vi "Send Message.vi"(7 "Data DVR":refnum<data-value>, 8 "Error In":errorcluster, 11 "Notify Only in":refnum<class "Notify Only.lvclass">) -> (0 "Error Out":errorcluster, 3 "Notify Only out":refnum<class "Notify Only.lvclass">)   [LabVIEW 2023, in "Notify Only.lvclass"]
uses:
  Notify Only.lvclass
  Data/Data.lvclass
  Controls/User Event Operations.ctl
  Notify Only.lvclass/Notify Only.ctl
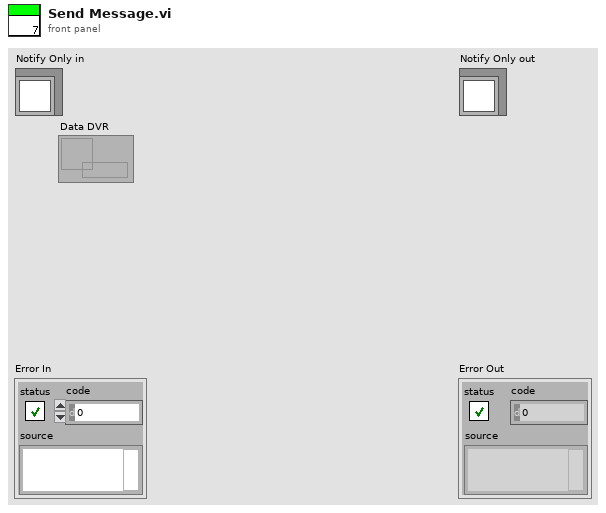
[diagram p1: front panel]
types:
  T1 = typedef "User Event Operations.ctl" = enum16{"Obtain", "Generate", "Destroy"}
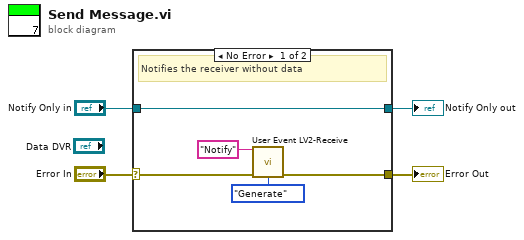
[diagram p0: block diagram]
diagram:
  n1 = case shown="No Error" "Error In" {
    selector: "Error In" -> [w6 w10]
    tunnel: [w5 w10] -> w3
    tunnel: [w9 w11] -> w1
    tunnel: "Notify Only in" -> [w9 w11]
    frame No Error {
      # "Notifies the receiver without data"
      n2 = call "User Event LV2-Receive.vi"("Event Name"="Notify", "Error In"=w6, "Operation"=User_Event_Operations."Generate") -> ("Error Out"=w5:errorcluster)  [unwired: 11 in, 1 out]
    }
    frame Error {
    }
  }
  "Error Out" <- w3
  "Notify Only out" <- w1
